vi "Set Car Wash Option Started Event.vi"(7 "Name":string, 10 "Format":string, 11 "Option":string) -> (3 "Car Wash Option Started out":refnum<class "Car Wash Option Started.lvclass">)   [LabVIEW 2016, in "CLD Exam - Car Wash.lvlib" / "Car Wash Option Started.lvclass"]
uses:
  Car Wash Option Started.lvclass
  D:/Repos/Stream/software/Mediator/Classes/Message Interface/Message Interface.lvclass
  Car Wash Option Started.lvclass/Car Wash Option Started.ctl
  Mediator/Classes/Message Interface/Message Interface.lvclass
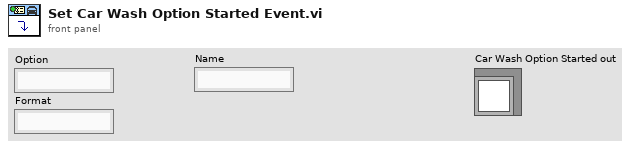
[diagram p1: front panel]
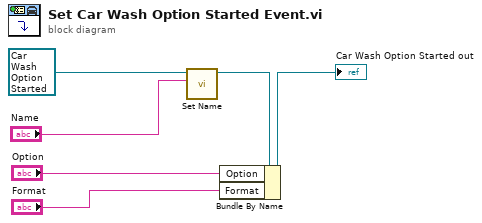
[diagram p0: block diagram]
diagram:
  n1 = call "Set Name.vi"("Name"="Name", "Message Interface in"=refnum<class "Car Wash Option Started.lvclass"> refnum ("Car Wash Option Started in")) -> ("Message Interface out"=w1:refnum<class "Car Wash Option Started.lvclass">)  [unwired: 8 in, 1 out]
  n2 = Bundle By Name(cluster=w1, "Option"="Option", "Format"="Format") -> (→"Car Wash Option Started out":refnum<class "Car Wash Option Started.lvclass">)
